vi "threshold.vi"(8 "Error in":errorcluster caption="Error in (no error)", 9 "Threshold Parameters (in)":T1, 10 "Threshold max (in)":i32, 11 "Threshold min (in)":i32) -> (0 "Error out":errorcluster, 1 "Threshold Parameters (out)":T1, 2 "Threshold max (out)":i32, 3 "Threshold min (out)":i32, 4 "Threshold Time (ms)":dbl)   [LabVIEW 2018]
uses:
  Controls/threshold_parameters.ctl
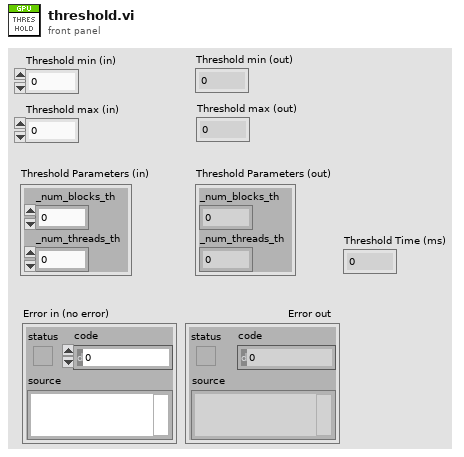
[diagram p1: front panel]
types:
  T1 = typedef "threshold_parameters.ctl" = cluster{"_num_blocks_th":i32, "_num_threads_th":i32}
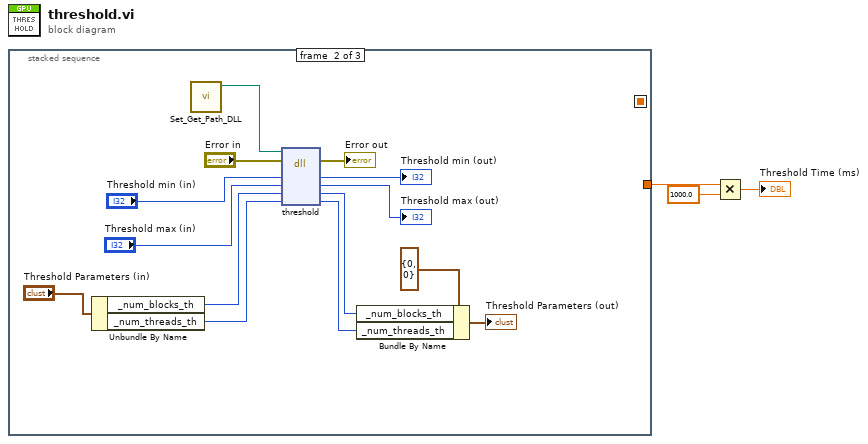
[diagram p0: block diagram]
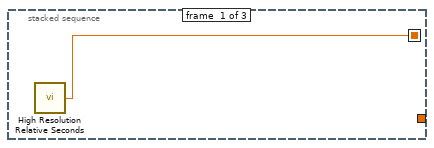
[diagram p2: hidden frame]
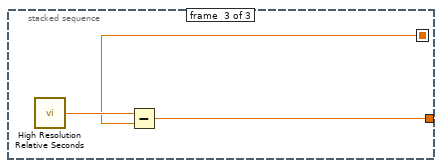
[diagram p3: hidden frame]
diagram:
  n1 = stacked-sequence {
    seq-local: [w4 _ _] -> [_ _ w20]
    tunnel: [_ _ w19] -> w1
    frame #0 {
      n2 = call <vilib>:"High Resolution Relative Seconds.vi"() -> ("relative seconds"=w4:dbl)
    }
    frame #1 {
      n3 = Unbundle By Name("Threshold Parameters (in)") -> ("_num_blocks_th"=w11:i32, "_num_threads_th"=w10:i32)
      n4 = call "Set_Get_Path_DLL.vi"() -> ("path DLL Out"=w5:path)  [unwired: 11 in]
      n5 = dll-call lib="C:/Users/AUTIS/Documents/TFG/Proyecto/Visual Studio/SR_GPU_TOOLKIT_INIT/x64/Release/SR_GPU_TOOLKIT.dll" fn="threshold"(path in=w5, error in="Error in", "min"="Threshold min (in)", "max"="Threshold max (in)", "_num_blocks_th"=w11, "_num_threads_th"=w10) -> (error out=→"Error out":errorcluster, "min"=→"Threshold min (out)":i32, "max"=→"Threshold max (out)":i32, "_num_blocks_th"=w7:i32, "_num_threads_th"=w6:i32)  [unwired: 2 in, 1 out]
      n6 = Bundle By Name(cluster=T1 {"_num_blocks_th"=0, "_num_threads_th"=0} ("Threshold Parameters (out)"), "_num_blocks_th"=w7, "_num_threads_th"=w6) -> (→"Threshold Parameters (out)":T1)
    }
    frame #2 {
      n7 = call <vilib>:"High Resolution Relative Seconds.vi"() -> ("relative seconds"=w21:dbl)
      n8 = Subtract(x=w21, y=w20) -> (x-y=w19:dbl)
    }
  }
  n9 = Multiply(x=w1, y=1000.0) -> (x*y=→"Threshold Time (ms)":dbl)
